vi "Transition Type.vi"(11 "State Transition Config in":refnum<class "State Transition Config.lvclass">) -> (2 "Transition Type":string)   [LabVIEW 2020, in "VolatusSeqConfig.lvlib" / "State Transition Config.lvclass"]
uses:
  State Transition Config.lvclass
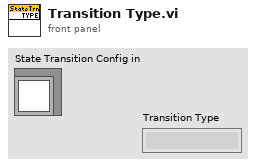
[diagram p1: front panel]
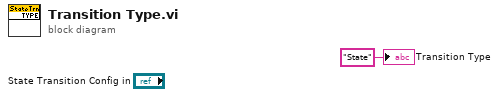
[diagram p0: block diagram]
diagram:
  "Transition Type" <- "State" ("Transition Type")
